vi "_VIVIs.vi"() -> (3 "Array":refnum<vi>[](array[refnum]))   [LabVIEW 2017, in "tagdb-UIStateExpr Operations.lvlib"]
uses:
  tagdb-UIStateExpr Operations.lvlib
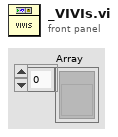
[diagram p1: front panel]
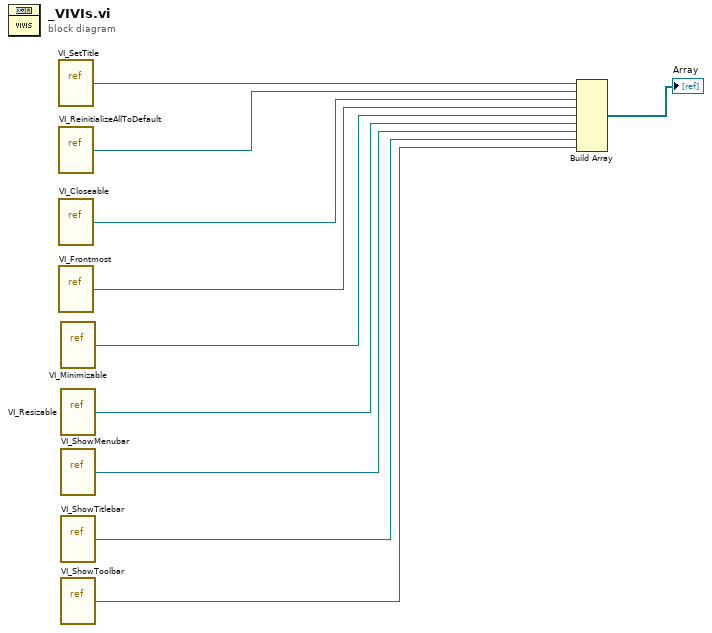
[diagram p0: block diagram]
diagram:
  n1 = vi-ref "VI_SetTitle.vi"() -> (w8:refnum<vi>)
  n2 = vi-ref "VI_ReinitializeAllToDefault.vi"() -> (w10:refnum<vi>)
  n3 = vi-ref "VI_Closeable.vi"() -> (w7:refnum<vi>)
  n4 = vi-ref "VI_Frontmost.vi"() -> (w6:refnum<vi>)
  n5 = vi-ref "VI_Minimizable.vi"() -> (w5:refnum<vi>)
  n6 = vi-ref "VI_Resizable.vi"() -> (w4:refnum<vi>)
  n7 = vi-ref "VI_ShowMenubar.vi"() -> (w3:refnum<vi>)
  n8 = vi-ref "VI_ShowTitlebar.vi"() -> (w2:refnum<vi>)
  n9 = vi-ref "VI_ShowToolbar.vi"() -> (w1:refnum<vi>)
  n10 = Build Array(w8, w10, w7, w6, w5, w4, w3, w2, w1) -> (→"Array":refnum<vi>[])
